vi "ManualThresholdLocalization-1.vi"(6 "[IN] Autothreshold Images \nInstead Of Generated U8":bool, 7 "[IN] Median Filter":bool, 8 "error IN":errorcluster, 10 "[IN] Binarized Image":T2, 11 "[IN] Source Image":T2) -> (0 "error OUT":errorcluster, 2 "[OUT] X,Y Coordinates":dbl[](array[numeric]))   [LabVIEW 2020]
uses:
  <vilib>/vision/Image Controls.llb/IMAQ Image.ctl
  <vilib>/vision/NI_Vision_Development_Module.lvlib
panel:
  in  "[IN] Settings":T1={"Objects"=0, "Threshold"=128, "Reject Border"=FALSE, "Fill Holes"=FALSE, "Min Object Size"=FALSE, "Min Size"=3, "Max Object Size"=FALSE, "Max Size"=100, "Show Search Area"=FALSE, "Show Center"=TRUE, "Show Bounding Box"=TRUE} {"Objects" items=["Bright Objects", "Dark Objects"]; "Threshold" min=1 max=999999999 step=1; "Max Size" min=1 max=999999999 step=1; "Min Size" min=1 max=999999999 step=1}
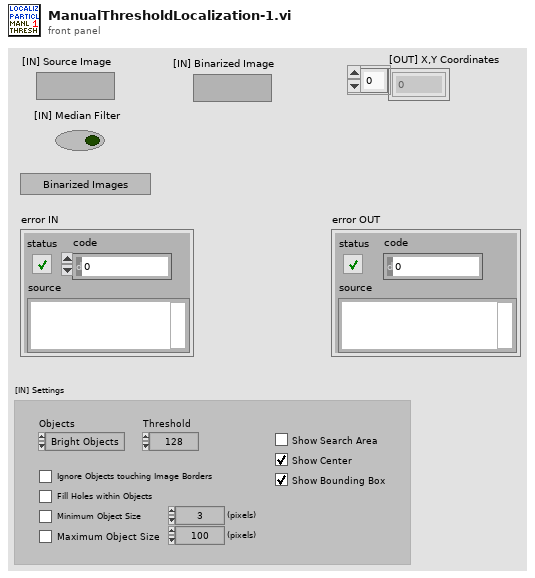
[diagram p1: front panel]
types:
  T1 = cluster{"Objects":u16, "Threshold":i32, "Reject Border":bool, "Fill Holes":bool, "Min Object Size":bool, "Min Size":i32, "Max Object Size":bool, "Max Size":i32, "Show Search Area":bool, "Show Center":bool, "Show Bounding Box":bool}
  T2 = typedef "IMAQ Image.ctl" = refnum<image>
  T3 = typedef "Image Type" = u32
  T4 = cluster{"X Size":i32, "Y Size":i32, "Order #":i32}
  T5 = cluster{"Object Center":cluster{"X":sgl, "Y":sgl}, "Bounding Box":cluster{"X Left":i32, "Y Top":i32, "X Right":i32, "Y Bottom":i32}, "Area":sgl, "Orientation":sgl, "Aspect Ratio":sgl, "Nb Holes":i32}[]
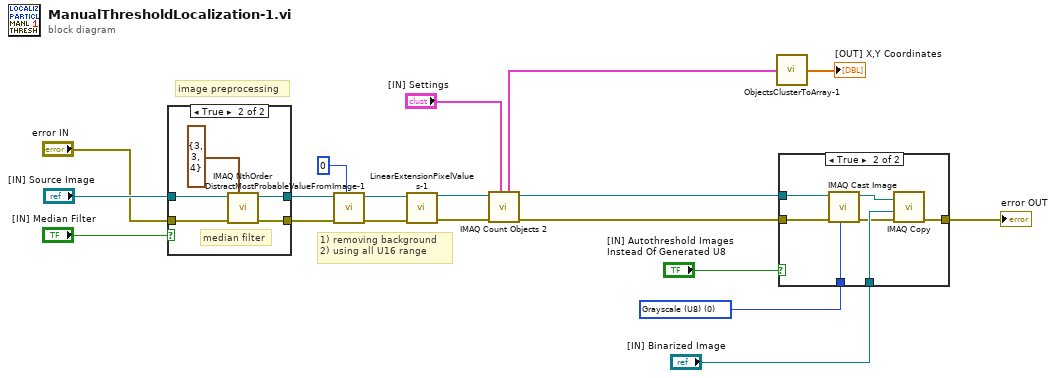
[diagram p0: block diagram]
diagram:
  w5 = T3 0 items=["Grayscale (U8)", "Grayscale (I16)", "Grayscale (SGL)", "Complex (CSG)", "RGB (U32)", "HSL (U32)", "RGB (U64)", "Grayscale (U16)"] ("Image Type")
  # "1) removing background\n2) using all U16 range"
  # "image preprocessing"
  n1 = case shown="True" "[IN] Median Filter" {
    tunnel: "[IN] Source Image" -> [w21 w25]
    tunnel: "error IN" -> [w20 w24]
    tunnel: [w21 w23] -> w15
    tunnel: [w20 w22] -> w14
    frame False {
    }
    frame True {
      # "median filter"
      n2 = call "IMAQ NthOrder"("Image Src"=w25, "Size & Order #"=T4 {"X Size"=3, "Y Size"=3, "Order #"=4}, "error in (no error)"=w24) -> ("Image Dst Out"=w23:T2, "error out"=w22:errorcluster)  [unwired: 4 in]
    }
  }
  n3 = call "DistractMostProbableValueFromImage-1.vi"("[IN] # Iteration"=0, "error in"=w14, "[IN] Max Projected Image"=w15) -> ("error out"=w11:errorcluster, "[OUT] Processed Image"=w12:T2)  [unwired: 6 in, 1 out]
  n4 = call "LinearExtensionPixelValues-1.vi"("error in"=w11, "[IN] Max Projected Image"=w12) -> ("error out"=w10:errorcluster, "[OUT] Processed Image"=w8:T2)  [unwired: 8 in]
  n5 = call "IMAQ Count Objects 2"("Settings"="[IN] Settings", "error in (no error)"=w10, "Image"=w8) -> ("error out"=w7:errorcluster, "Image Out"=w6:T2, "Objects"=w2:T5)  [unwired: 4 in, 2 out]
  n6 = call "ObjectsClusterToArray-1.vi"("[IN] Objects"=w2) -> ("[OUT] X,Y Coordinates"=→"[OUT] X,Y Coordinates":dbl[])
  n7 = case shown="True" "[IN] Autothreshold Images \nInstead Of Generated U8" {
    tunnel: w7 -> [w27 w33]
    tunnel: [w27 w34] -> w3
    tunnel: w6 -> [_ w32]
    tunnel: w5 -> [_ w31]
    tunnel: "[IN] Binarized Image" -> [_ w29]
    frame False {
    }
    frame True {
      n8 = call "IMAQ Cast Image"("Image Type"=w31, "error in (no error)"=w33, "Image Src"=w32) -> ("error out"=w28:errorcluster, "Image Dst Out"=w30:T2)  [unwired: 7 in]
      n9 = call "IMAQ Copy"("error in (no error)"=w28, "Image Dst"=w29, "Image Src"=w30) -> ("error out"=w34:errorcluster)  [unwired: 3 in, 1 out]
    }
  }
  "error OUT" <- w3
